vi "GetBuvCurrent (SubVI).vi"(0 "connection ID in":refnum<k5>, 5 "error in":errorcluster) -> (8 "Buv I":string, 14 "connection ID out":refnum<k5>, 19 "error out":errorcluster)   [LabVIEW 2013]
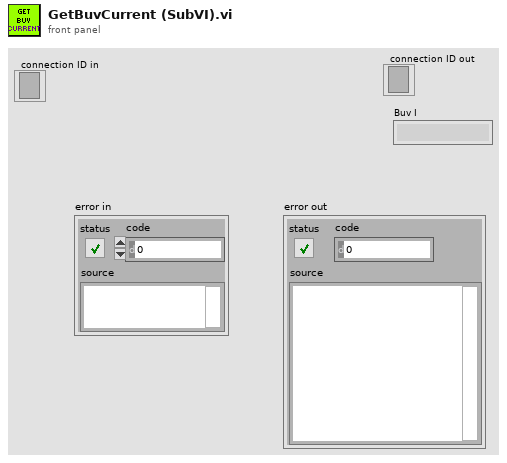
[diagram p1: front panel]
types:
  T1 = enum16{"Standard", "Buffered", "CRLF", "Immediate"}
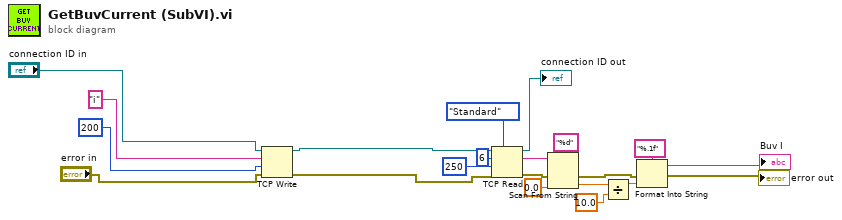
[diagram p0: block diagram]
diagram:
  n1 = TCP Write(connection ID="connection ID in", data in="i", error in (no error)="error in", 9:200 ("timeout ms (25000)")) -> (connection ID out=w2:refnum<k5>, error out=w1:errorcluster)  [unwired: 1 out]
  n2 = TCP Read(connection ID=w2, bytes to read=6, error in (no error)=w1, 7:T1."Standard" ("mode (standard)"), 9:250 ("timeout ms (25000)")) -> (connection ID out=→"connection ID out":refnum<k5>, data out=w17:string, error out=w14:errorcluster)
  n3 = Scan From String(format string="%d", input string=w17, error in=w14, default 1=0.0 ("default value 1")) -> (error out=w3:errorcluster, output 1=w7:dbl)  [unwired: 1 in, 2 out]
  n4 = Divide(x=w7, y=10.0) -> (x/y=w5:dbl)
  n5 = Format Into String(format string="%.1f", error in=w3, w5) -> (resulting string=→"Buv I":string, error out=→"error out":errorcluster)  [unwired: 1 in]
